vi "NewAutoGlobals.vi"() -> ()   [LabVIEW 2023]
uses:
  NewAutoStepTypeEnum.ctl
  NewAutoStepTypedef.ctl
panel:
  in  "NewAuto030":T1[](array[typedef])
  in  "NewAuto029":T1[](array[typedef])
  in  "NewAuto028":T1[](array[typedef])
  in  "NewAuto027":T1[](array[typedef])
  in  "NewAuto026":T1[](array[typedef])
  in  "NewAuto025":T1[](array[typedef])
  in  "NewAuto024":T1[](array[typedef])
  in  "NewAuto023":T1[](array[typedef])
  in  "NewAuto022":T1[](array[typedef])
  in  "NewAuto021":T1[](array[typedef])
  in  "NewAuto020":T1[](array[typedef])
  in  "NewAuto019":T1[](array[typedef])
  in  "NewAuto018":T1[](array[typedef])
  in  "NewAuto017":T1[](array[typedef])
  in  "NewAuto016":T1[](array[typedef])
  in  "NewAuto015":T1[](array[typedef])
  in  "NewAuto014":T1[](array[typedef])
  in  "NewAuto013":T1[](array[typedef])
  in  "NewAuto012":T1[](array[typedef])
  in  "NewAuto011":T1[](array[typedef])
  in  "NewAuto010":T1[](array[typedef])
  in  "NewAuto009":T1[](array[typedef])
  in  "NewAuto008":T1[](array[typedef])
  in  "NewAuto007":T1[](array[typedef])
  in  "NewAuto006":T1[](array[typedef])
  in  "NewAuto005":T1[](array[typedef])
  in  "NewAuto004":T1[](array[typedef])
  in  "NewAuto003":T1[](array[typedef])
  in  "NewAuto002":T1[](array[typedef])
  in  "NewAuto001":T1[](array[typedef])
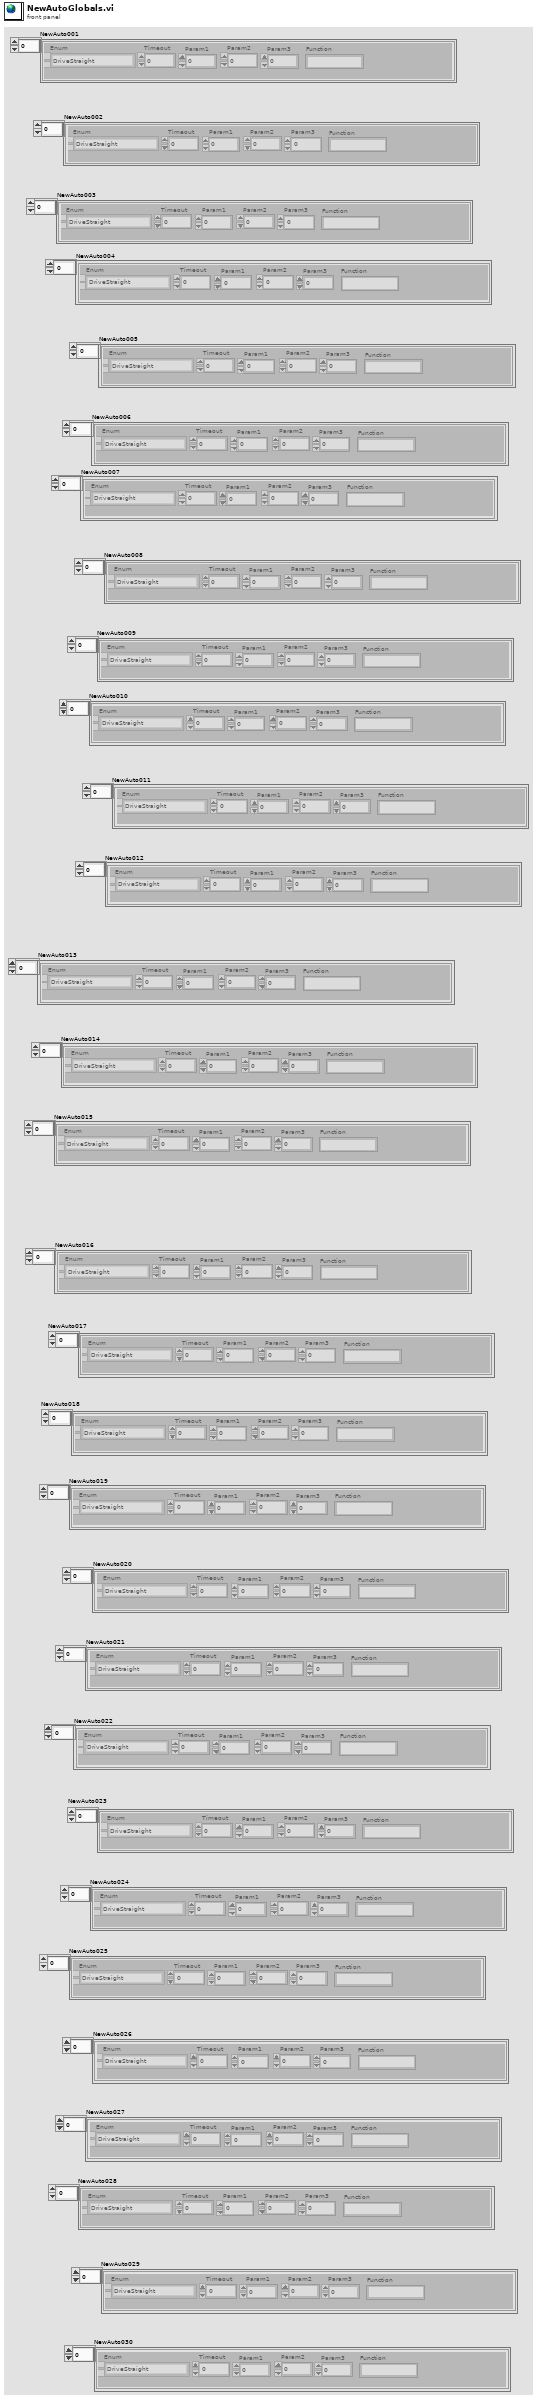
[diagram p1: front panel]
types:
  T1 = typedef "NewAutoStepTypedef.ctl" = cluster{"Enum":T2, "Timeout":dbl, "Param1":dbl, "Param2":dbl, "Param3":dbl, "Function":string}
  T2 = typedef "NewAutoStepTypeEnum.ctl" = enum16{"DriveStraight", "DriveTurn", "FollowAbsoluteTrajectory", "FollowRelativeTrajectory", "AutoWait", "ElevToRest", "ElevToFloor", "ElevToSource", "ElevToL1", "ElevToL2", "ElevToL3", "ElevToL4", "ElevToAlgae1", "ElevToAlgae2", "ElevToBarge", "ElevCancel", "IntakeCoral", "IntakeAlgae", "IntakeDepositCoral", "IntakeDepositAlgae", "IntakeCancel", "ElevRestWait", "ElevFloorWait", "ElevSourceWait", "ElevL1Wait", "ElevL2Wait", "ElevAlgae1Wait", "ElevL3Wait", "ElevAlgae2Wait", "ElevL4Wait", "ElevBargeWait"}
diagram:
